vi "ErrorMSG_UI.vi"() -> ()   [LabVIEW 2019]
uses:
  <vilib>/Utility/miscctls.llb/LVPositionTypeDef.ctl
  <vilib>/Utility/miscctls.llb/LVPointTypeDef.ctl
  Ctrl/AlarmReportCtrl.ctl
  Class/Main Process Class/MPC_AutoPaste/Ctrl/ModbusCmd.ctl
  Class/Main Process Class/MPC_AutoPaste/Ctrl/Auto Inspection Station Name2.ctl
  Class/Main Process Class/MPC_AutoPaste/Ctrl/Auto Inspection Data Name.ctl
  IO Folder/IO_VI/IOCtrl/Ctrl/64Out_2 SelectOut.ctl
  0d8d3c4f-70c5-4d62-a714-a7cb91084a9f.vi
  Global/ErrorMsg_LinkData.vi
  LLB/Commonly VI/Main Glb.vi
  <vilib>/JDP Science/JSONtext/JSON text to Variant.vi
  LLB/Commonly VI.lvlib
panel:
  out "PanelOff":bool=TRUE
  out "ErrResetFlg":bool=TRUE
  in  "Tab Error":enum32{"Page 1", "Page 2"}(tab)
  out "Error List":i32(listbox)
  in  "Error Reset":bool
  in  "Buzzer Stop":bool
  out "Warning List":i32(listbox)
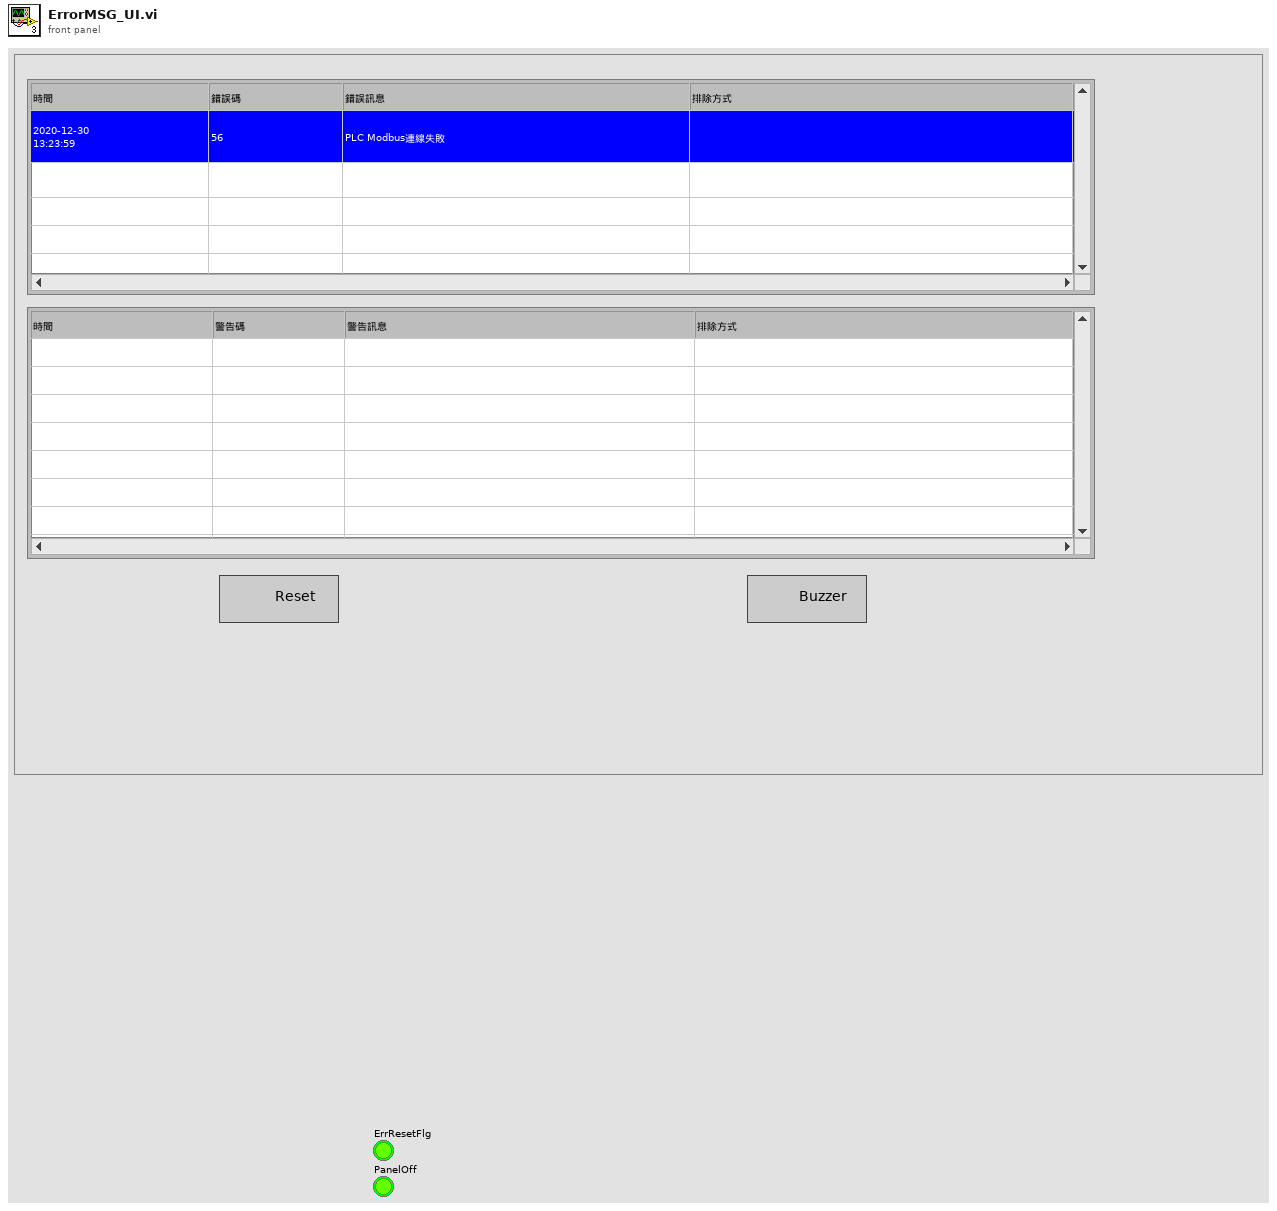
[diagram p1: front panel]
types:
  T1 = typedef "LVPointTypeDef.ctl" = cluster{"Horizontal":i16, "Vertical":i16}
  T2 = typedef "LVPositionTypeDef.ctl" = cluster{"Left":i32, "Top":i32}
  T3 = typedef "AlarmReportCtrl.ctl" = enum16{"Initial", "AddError", "WriteAlarmResetTime", "WriteOPID", "Load", "Save", "WriteRootCause"}
  T4 = cluster{"starting address":u16, "number of inputs":u16, "Sat Coils":bool[], "Holding Registers":u16[]}
  T5 = typedef "ModbusCmd.ctl" = enum16{"Connect", "Disconnect", "Init", "Fetch Basic Objects", "Fetch Input Refisters", "Fetch Discrete Inputs", "Set Coils", "Set Holding Registers", "Write Single Holding", "Exit"}
  T6 = enum16{"idle", "error occurs", "warning occurs", "error cleared", "warning cleared", "run"}
  T7 = typedef "Auto Inspection Data Name.ctl" = enum16{"LocalRun", "ItemSN(TimeCode)", "CurrentAction", "Error", "Data", "OKNG", "電壓值", "電壓值判斷", "電流值", "電流值判斷", "Laser1 Data", "Laser2 Data", "Laser OKNG", "StationNO"}
  T8 = typedef "64Out_2 SelectOut.ctl" = enum16{"移入軌道氣缸#模組七", "軌道分料氣缸#模組七", "移入旋轉台氣缸#模組七", "旋轉台氣缸#模組七", "收料燈號#模組七", "UBE#2", "汽缸升_1#移載一", "汽缸降_1#移載一", "汽缸升_2#移載一", "汽缸降_2#移載一", "放料汽缸_1#移載一", "放料汽缸_2#移載一", "汽缸升_3#移載二", "汽缸降_3#移載二", "汽缸升_4#移載二", "汽缸降_4#移載二", "放料汽缸_3#移載二", "放料汽缸_4#移載二", "汽缸升_5#移載三", "汽缸降_5#移載三", "汽缸升_6#移載三", "汽缸降_6#移載三", "放料汽缸_5#移載三", "放料汽缸_6#移載三", "汽缸升_7#移載四", "汽缸降_7#移載四", "放料汽缸_7#移載四", "UBE#10", "綠", "黃", "紅", "嗡鳴器", "UBE#15", "UBE#16", "UBE#17", "UBE#18", "UBE#19", "UBE#20", "UBE#21", "UBE#22", "UBE#23", "UBE#24", "UBE#25", "UBE#26", "UBE#27", "UBE#28", "UBE#29", "UBE#30", "UBE#31", "UBE#32", "UBE#33", "UBE#34", "UBE#35", "UBE#36", "UBE#37", "UBE#38", "UBE#39", "UBE#40", "UBE#41", "UBE#42", "UBE#43", "UBE#44", "UBE#45", "UBE#46"}
  T9 = cluster{"status":bool, "Error Code":i32, "String":string}
  T10 = typedef "Auto Inspection Station Name2.ctl" = enum16{"S1Barcode", "S2Measure", "S3Measure", "S4Measure", "S5Measure", "S11_LaserCheck", "S8_Vision AI"}
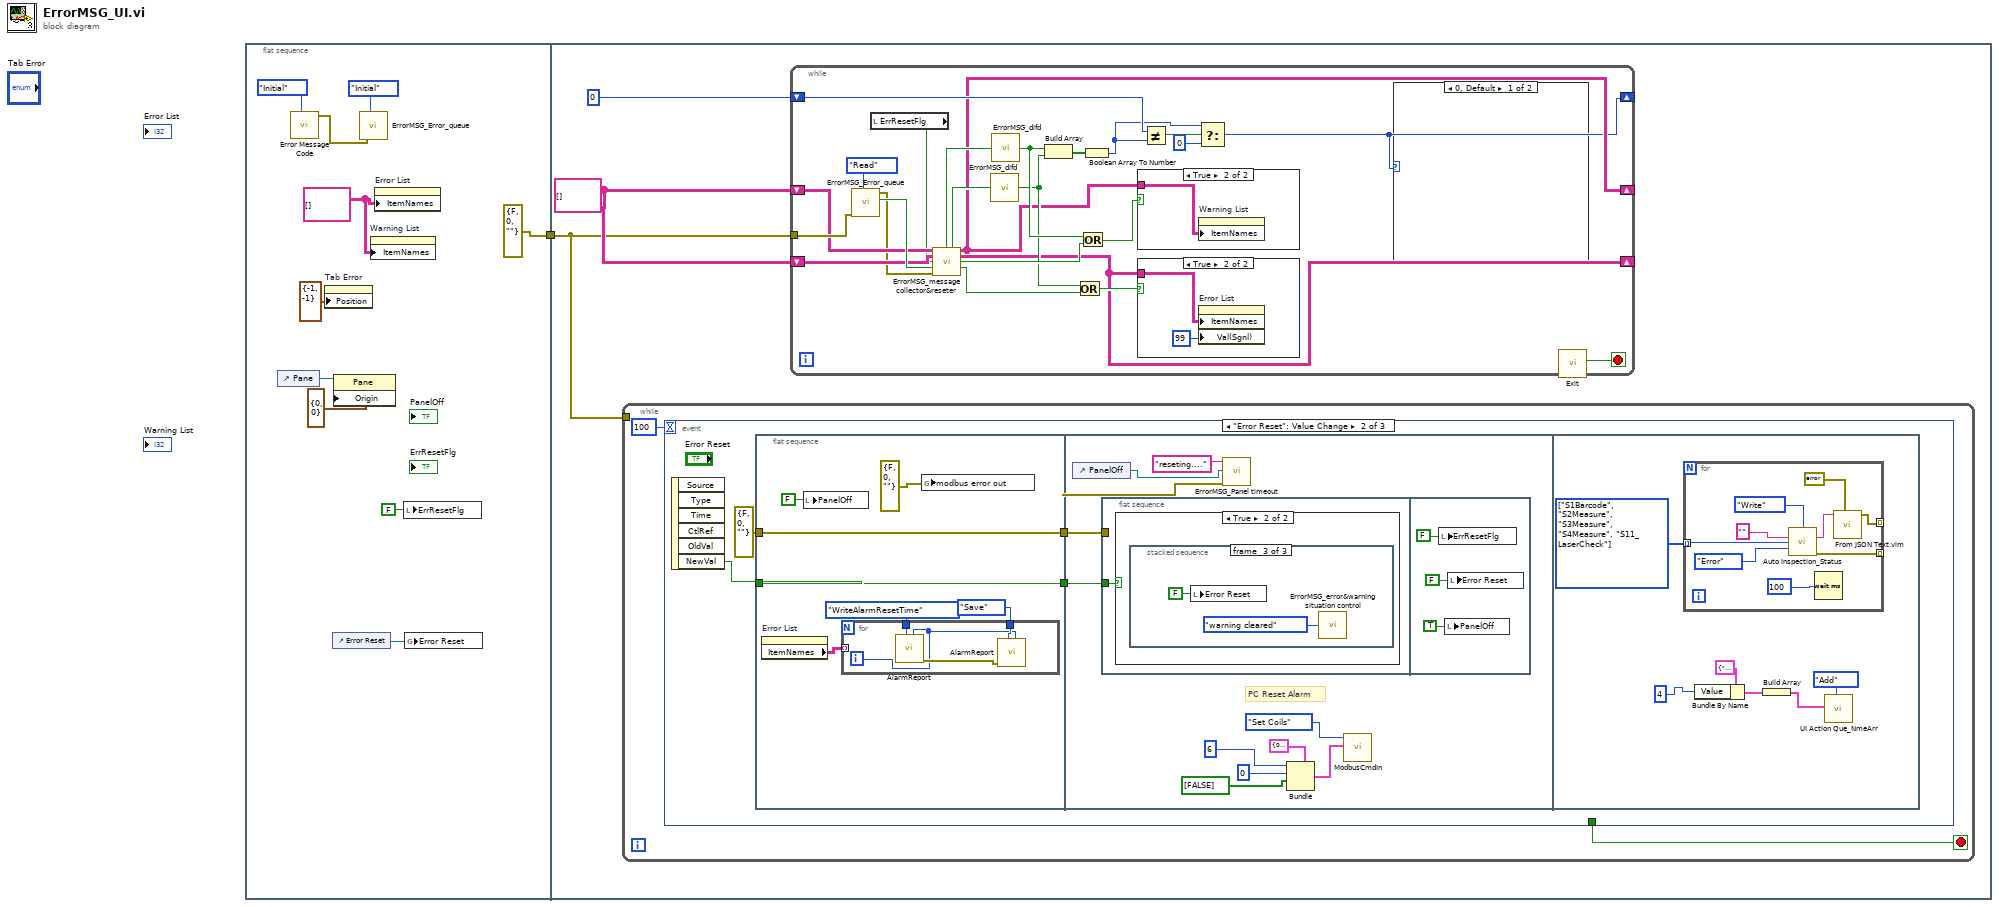
[diagram p0: block diagram]
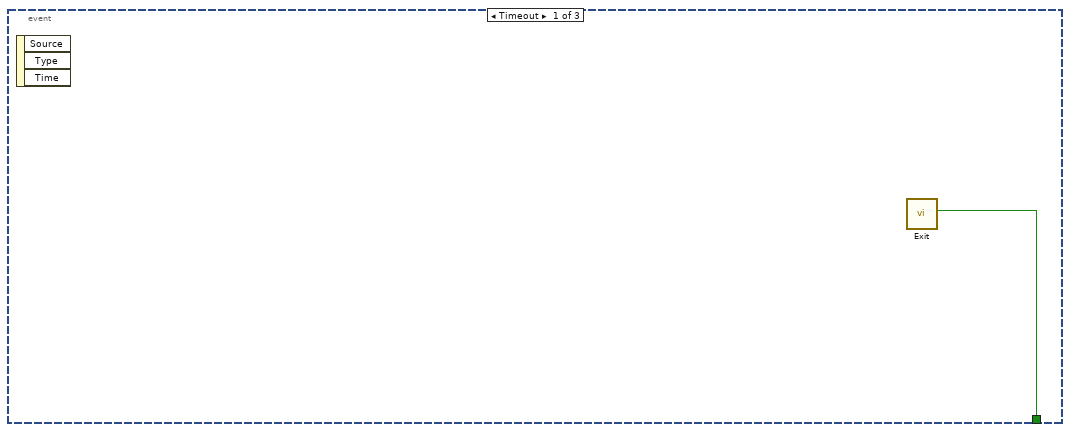
[diagram p2: hidden frame]
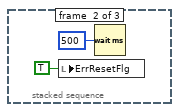
[diagram p5: hidden frame]
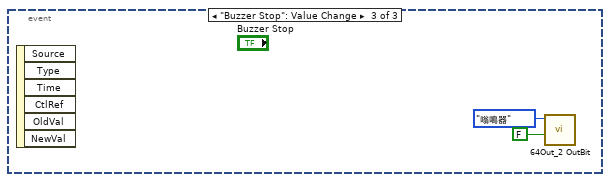
[diagram p6: hidden frame]
diagram:
  n1 = flat-sequence {
    tunnel: [errorcluster {"status"=FALSE, "code"=0, "source"=""} ("error in (no error)")] -> w1
    tunnel: w1 -> [w12]
    frame #0 {
      w9 = string[][] []
      n2 = control-ref of="Pane"() -> (w8:refnum<vi>)
      n3 = call "Error Message Code.vi"("Enum"=enum16{"Initial", "ErrorIn"}."Initial") -> ("Error Message"=w2:T9)  [unwired: 10 in]
      n4 = property on="Tab Error" class="TabCtl (strict)"("Position"=T2 {"Left"=-1, "Top"=-1}) -> ()  [unwired: 2 in, 2 out]
      n5 = control-ref of="Error Reset"() -> (w3:refnum<vi>)
      n6 = property class="Pane"(reference=w8, "Origin"=T1 {"Horizontal"=0, "Vertical"=0}) -> ()  [unwired: 1 in, 2 out]
      n7 = call "ErrorMSG_Error_queue.vi"("Method"=enum16{"Initial", "Add", "Read", "Delete"}."Initial", "error in (no error)"=w2) -> ()  [unwired: 7 in, 3 out]
      n8 = property on="Warning List" class="MCListbox (strict)"("ItemNames"=w9) -> ()  [unwired: 2 in, 2 out]
      n9 = property on="Error List" class="MCListbox (strict)"("ItemNames"=w9) -> ()  [unwired: 2 in, 2 out]
      n10 = local write "ErrResetFlg"(FALSE ("ErrResetFlg")) -> ()
      n11 = global write "ErrorMsg_LinkData.vi" "Error Reset"(w3) -> ()
    }
    frame #1 {
      w14 = string[][] []
      n12 = while {
        tunnel: w12 -> [_]
        stop <- w16 stop-if-true
        n13 = event shown="[1] \"Error Reset\": Value Change" {
          selector: _ -> [_ _ _]
          dyn-events: _ -> [_ _ _]
          timeout: 100 -> [_ _ _]
          tunnel: [w17 _ _] -> w16
          event Timeout {
            n14 = event-data() -> ()  [unwired: 1 in, 3 out]
            n15 = call "Exit.vi"() -> ("ExitOut"=w17:bool)  [unwired: 11 in]
          }
          event "Error Reset": Value Change {
            n16 = event-data() -> ("NewVal"=w21:bool)  [unwired: 1 in, 5 out]
            n17 = flat-sequence {
              tunnel: errorcluster {"status"=FALSE, "code"=0, "source"=""} ("error constant") -> [w27]
              tunnel: w21 -> [w28]
              tunnel: [w28] -> w19
              tunnel: [w27] -> w18
              tunnel: w19 -> [w42]
              tunnel: w18 -> [w40]
              frame #0 {
                n18 = property on="Error List" class="MCListbox (strict)"() -> ("ItemNames"=w24:string[][])  [unwired: 2 in, 2 out]
                n19 = local write "PanelOff"(FALSE ("PanelOff")) -> ()
                n20 = for {
                  tunnel: AlarmReportCtrl."WriteAlarmResetTime" ("Emun") -> [w32]
                  tunnel: w24 -> [_] mode=indexing
                  tunnel: AlarmReportCtrl."Save" ("Emun") -> [w31]
                  i -> [w29]
                  n21 = call "AlarmReport.vi"("PalletError"=w29, "Emun"=w32) -> ("error out"=w30:errorcluster)  [unwired: 9 in]
                  n22 = call "AlarmReport.vi"("PalletError"=w29, "Emun"=w31, "VILinkerror In"=w30) -> ()  [unwired: 8 in, 1 out]
                }
                n23 = global write "Main Glb.vi" "modbus error out"(errorcluster {"status"=FALSE, "code"=0, "source"=""} ("modbus error out")) -> ()
              }
              frame #1 {
                # "PC Reset Alarm"
                n24 = control-ref of="PanelOff"() -> (w39:refnum<vi>)
                n25 = flat-sequence {
                  tunnel: w40 -> [_]
                  tunnel: w42 -> [w43]
                  frame #0 {
                    n26 = case shown="True" w43 {
                      frame False {
                      }
                      frame True {
                        n27 = stacked-sequence {
                          frame #0 {
                          }
                          frame #1 {
                            n28 = local write "ErrResetFlg"(TRUE ("ErrResetFlg")) -> ()
                            n29 = Wait (ms)(milliseconds to wait=u32 500) -> ()  [unwired: 1 out]
                          }
                          frame #2 {
                            n30 = local write "Error Reset"(FALSE ("Error Reset")) -> ()
                            n31 = call "ErrorMSG_error&warning situation control.vi"("error&warning control"=T6."warning cleared") -> ()  [unwired: 2 in]
                          }
                        }
                      }
                    }
                  }
                  frame #1 {
                    n32 = local write "ErrResetFlg"(FALSE ("ErrResetFlg")) -> ()
                    n33 = local write "PanelOff"(TRUE ("PanelOff")) -> ()
                    n34 = local write "Error Reset"(FALSE ("Error Reset")) -> ()
                  }
                }
                n35 = call "ErrorMSG_Panel timeout.vi"("error in (no error)"=w40, "reference"=w39, "String"="reseting....") -> ()  [unwired: 7 in, 2 out]
                n36 = Bundle(cluster=T4 {"starting address"=0, "number of inputs"=0, "Sat Coils"=[], "Holding Registers"=[]} ("data"), "starting address"=6, "number of inputs"=u16 0, "Sat Coils"=bool[] [FALSE]) -> (w38:T4)  [unwired: 1 in]
                n37 = call "ModbusCmdIn.vi"("data"=w38, "Enum"=ModbusCmd."Set Coils") -> ()  [unwired: 9 in, 1 out]
              }
              frame #2 {
                w56 = T10[] [enum."S1Barcode", enum."S2Measure", enum."S3Measure", enum."S4Measure", enum."S11_LaserCheck"] items=["S1Barcode", "S2Measure", "S3Measure", "S4Measure", "S5Measure", "S11_LaserCheck", "S8_Vision AI"]
                n38 = for {
                  tunnel: w56 -> [w64] mode=indexing
                  tunnel: [w63] -> _ mode=indexing
                  tunnel: [w58] -> _ mode=indexing
                  n39 = call "Auto Inspection_Status.vi"("Action"=enum16{"Initial", "Write", "Read"}."Write", "DataIn"="", "Station"=w64, "Data"=Auto_Inspection_Data_Name."Error") -> ("DataOut"=w60:string, "error out"=w63:errorcluster)  [unwired: 9 in, 1 out]
                  n40 = Wait (ms)(milliseconds to wait=100) -> ()  [unwired: 1 out]
                  n41 = call "From JSON Text.vim"("Data Type and Default Value"=errorcluster {"status"=FALSE, "code"=0, "source"=""} ("error constant"), "JSON"=w60) -> ("Data out"=w58:errorcluster)  [unwired: 8 in, 1 out]
                }
                n42 = Bundle By Name(cluster=cluster{"Action":string, "Value":variant} {"Action"="ChangePage", "Value"=variant} ("UI Action"), "Value"=4) -> (w54:cluster{"Action":string, "Value":variant})
                n43 = Build Array(w54) -> (w51:cluster{"Action":string, "Value":variant}[])
                n44 = call "UI Action Que_NmeArr.vi"("Action"=enum16{"Initial", "Add", "Release"}."Add", "UI Process"=w51) -> ()  [unwired: 8 in, 2 out]
              }
            }
          }
          event "Buzzer Stop": Value Change {
            n45 = event-data() -> ()  [unwired: 1 in, 6 out]
            n46 = call "64Out_2 OutBit.vi"("BL"=FALSE, "IO_Output_2 Select"=64Out_2_SelectOut."嗡鳴器") -> ()  [unwired: 9 in, 1 out]
          }
        }
      }
      n47 = while {
        tunnel: w12 -> [w91]
        shift-right: [w72] -> _
        shift-left: w14 -> [w88]
        shift-right: [w71] -> _
        shift-left: w14 -> [w87]
        shift-right: [w70] -> _
        shift-left: u32 0 ("f") -> [w77]
        stop <- w68 stop-if-true
        n48 = call "ErrorMSG_Error_queue.vi"("Method"=enum16{"Initial", "Add", "Read", "Delete"}."Read", "error in (no error)"=w91) -> ("timed out?"=w89:bool, "dequeue element"=w86:errorcluster)  [unwired: 7 in, 1 out]
        n49 = local read "ErrResetFlg"() -> (w69:bool)
        n50 = call "ErrorMSG_message collector&reseter.vi"("Warning List in"=w88, "Error List in"=w87, "Error reset"=w69, "dequeue timeout"=w89, "error &rester in"=w86) -> ("Warning Clear?"=w85:bool, "Error Clear"=w84:bool, "Warning List out"=w72:string[][], "Error List out"=w71:string[][], "Warning Expanded"=w82:bool, "Error Expanded"=w80:bool)  [unwired: 5 in]
        n51 = call "ErrorMSG_difd.vi"("input"=w84) -> ("output"=w81:bool)
        n52 = call "ErrorMSG_difd.vi"("input"=w85) -> ("output"=w83:bool)
        n53 = Build Array(w83, w81) -> (w78:bool[])
        n54 = Or(x=w81, y=w80) -> (x .or. y?=w79:bool)
        n55 = Or(x=w83, y=w82) -> (x .or. y?=w73:bool)
        n56 = Boolean Array To Number(Boolean array=w78) -> (number=w75:u32)
        n57 = case shown="True" w73 {
          tunnel: w72 -> [_ w92]
          frame False {
          }
          frame True {
            n58 = property on="Warning List" class="MCListbox (strict)"("ItemNames"=w92) -> ()  [unwired: 2 in, 2 out]
          }
        }
        n59 = case shown="True" w79 {
          tunnel: w71 -> [_ w94]
          frame False {
          }
          frame True {
            n60 = property on="Error List" class="MCListbox (strict)"("ItemNames"=w94, "Val(Sgnl)"=99 ("Value (Signaling)")) -> ()  [unwired: 2 in, 2 out]
          }
        }
        n61 = Not Equal?(x=w77, y=w75) -> (x != y?=w76:bool)
        n62 = Select(t=w75, s=w76, f=u32 0) -> (s? t:f=w70:u32)
        n63 = case shown="0, Default" w70 {
          frame 0, Default {
          }
          frame 1 {
          }
        }
        n64 = call "Exit.vi"() -> ("ExitOut"=w68:bool)  [unwired: 11 in]
      }
    }
  }
